vi "Create or Close PDFReader.vi"(2 "Action":T1, 5 "PdfReader IN":refnum<k24>, 7 "PDF File and position":T2={"Path"=path "", "Pages"="all", "Source"=enum."File to add", "Start at page old"=0, "Start at page new"=1, "Owner password"=""}, 11 "error in (no error)":errorcluster) -> (4 "PDFReaderIsOpen?":bool, 6 "PdfReader OUT":refnum<k24>, 8 "NumberOfPages":i32, 10 "Page [ ]":i32[](array[numeric]), 15 "error out":errorcluster)   [LabVIEW 2019, in "Exaprom PDF.lvlib"]
doc: "Version 1.1\nDeveloped by Jean-Marc Simard\nCopyright © 2012, Exaprom Inc.\nAll rights reserved.\nLicense: BSD\n\nWith iTextSharp 4.1.6 (http://itextsharp.sourceforge.net)\nunder Mozilla Public License Version 1.1\n(http://www.mozilla.org/MPL/MPL-1.1.html)"
uses:
  Controls/Concatenate Controls/PDF File and position.ctl
  Controls/Concatenate Controls/PDF file source.ctl
  C:/work/niobrara_lv/labview pdf writer fixing/DLL/itextsharp.dll
  DLL/itextsharp.dll
  Controls/General Controls/Create or close.ctl
  Exaprom PDF.lvlib
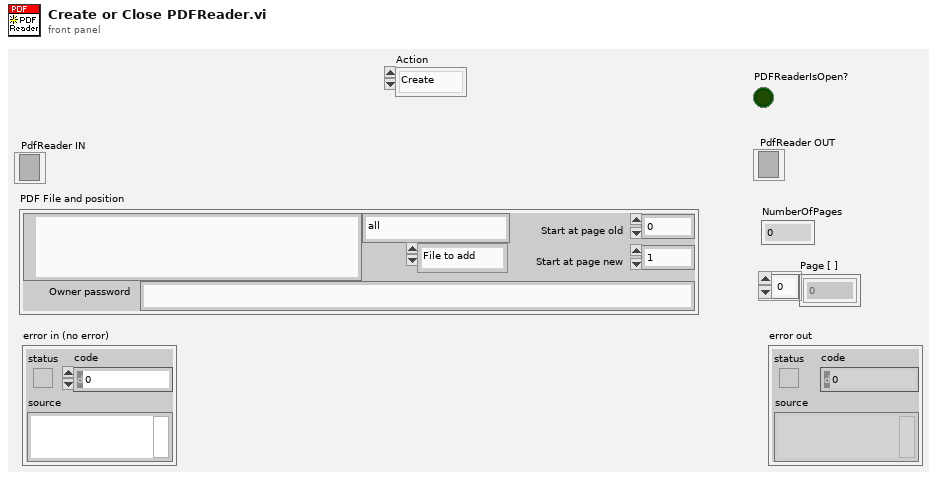
[diagram p1: front panel]
types:
  T1 = typedef "Exaprom PDF.lvlib/Create or close.ctl" = enum16{"Create", "Close"}
  T2 = typedef "Exaprom PDF.lvlib/PDF File and position.ctl" = cluster{"Path":path, "Pages":string, "Source":T3, "Start at page old":i32, "Start at page new":i32, "Owner password":string}
  T3 = typedef "Exaprom PDF.lvlib/PDF file source.ctl" = enum16{"PDF Report", "File to add"}
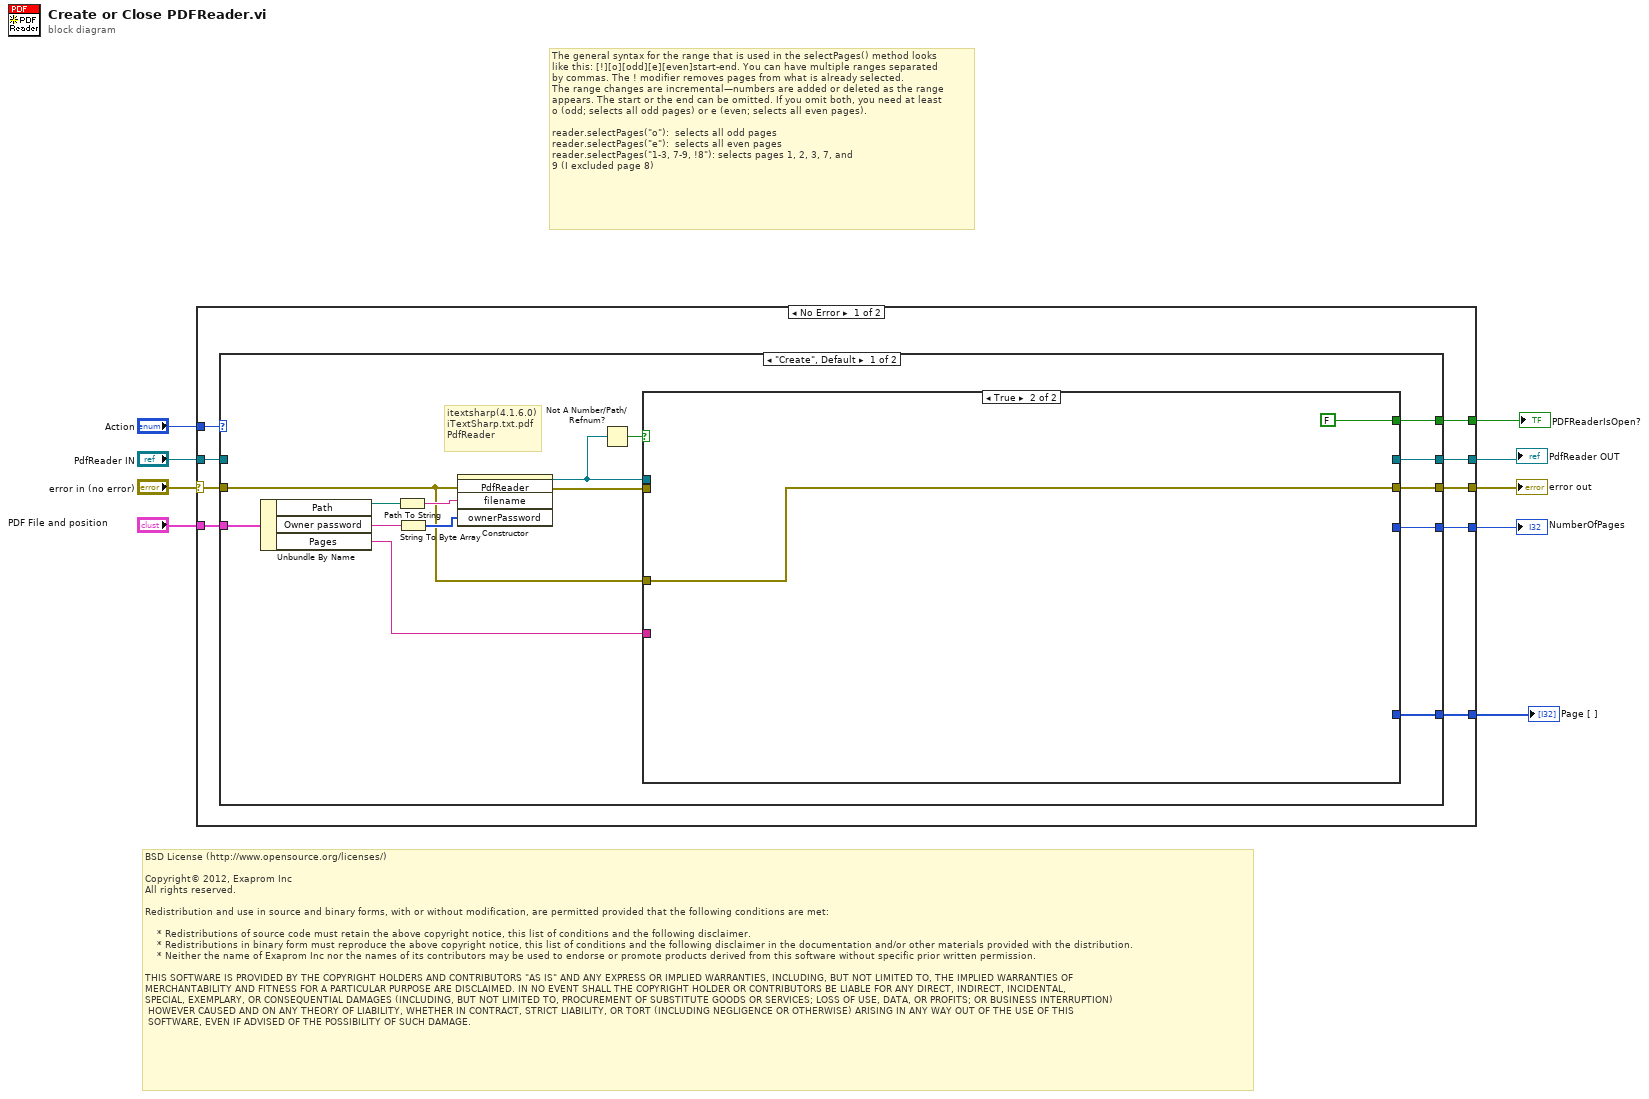
[diagram p0: block diagram]
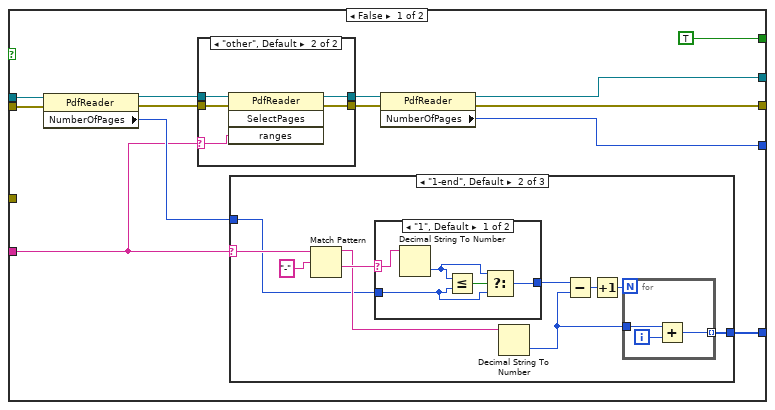
[diagram p2: hidden frame]
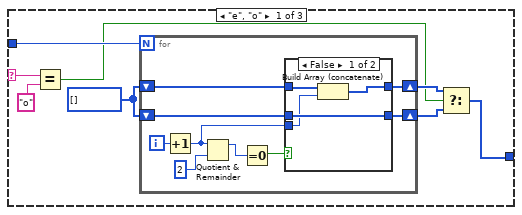
[diagram p3: hidden frame]
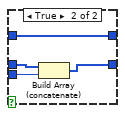
[diagram p4: hidden frame]
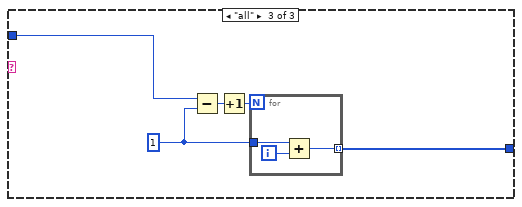
[diagram p6: hidden frame]
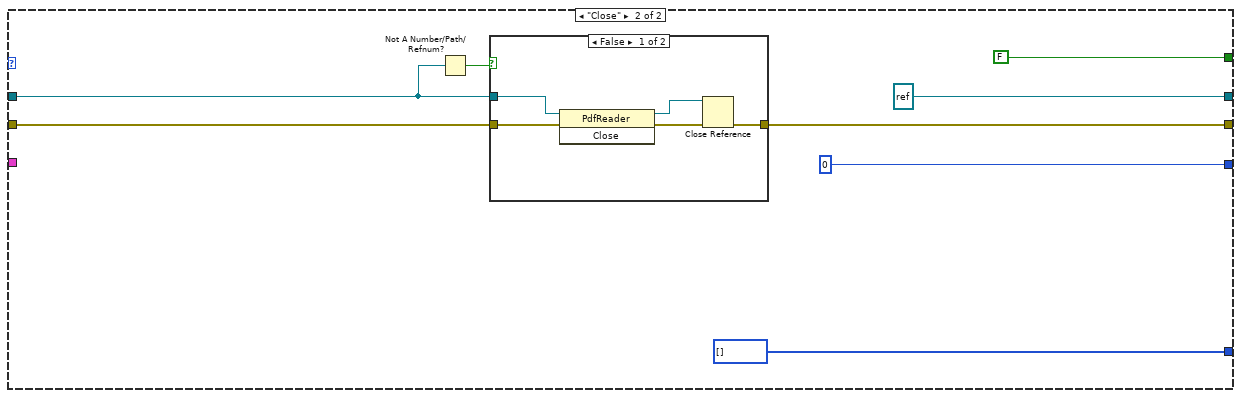
[diagram p8: hidden frame]
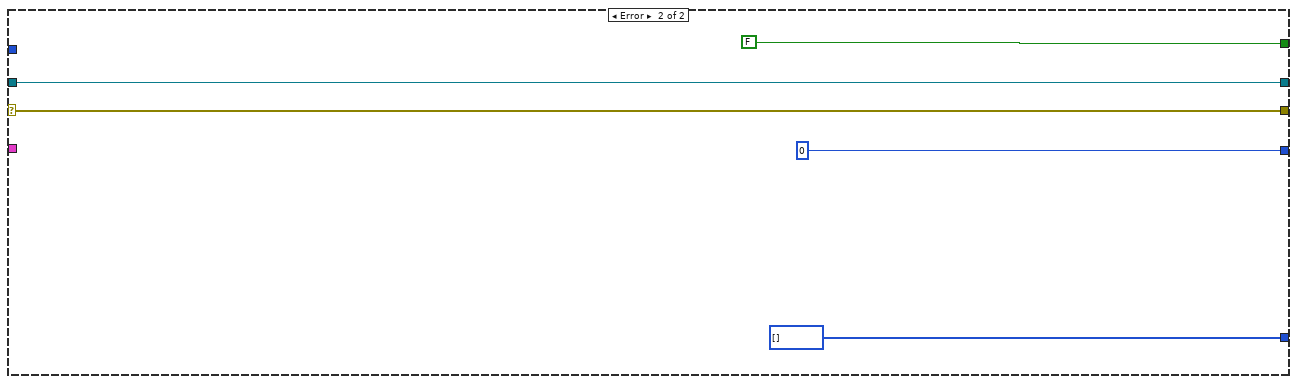
[diagram p10: hidden frame]
diagram:
  # "The general syntax for the range that is used in the selectPages() method looks\nlike this: [!][o][odd][e][even]start-end. You can have multiple ranges separated\nby commas. The ! modifier removes pages from what is already selected.\nThe range changes are incremental—numbers are added or deleted as the range\nappears. The start or the end can be omitted. If you omit both, you need at least\no (odd; selects all odd pages) or e (even; selects all even pages).\n\nreader.selectPages(\"o\"):  selects all odd pages\nreader.selectPages(\"e\"):  selects all even pages\nreader.selectPages(\"1-3, 7-9, !8\"): selects pages 1, 2, 3, 7, and\n9 (I excluded page 8)"
  # "BSD License (http://www.opensource.org/licenses/)\n\nCopyright© 2012, Exaprom Inc\nAll rights reserved.\n\nRedistribution and use in source and binary forms, with or without modification, are permitted provided that the following conditions are met:\n\n    * Redistributions of source code must retain the above copyright notice, this list of conditions and the following disclaimer.\n    * Redistributions in binary form must reproduce the above copyright notice, this list of conditions and the following disclaimer in the documentation and/or other materials provided with the distribution.\n    * Neither the name of Exaprom Inc nor the names of its contributors may be used to endorse or promote products derived from this software without specific prior written permission.\n\nTHIS SOFTWARE IS PROVIDED BY THE COPYRIGHT HOLDERS AND CONTRIBUTORS \"AS IS\" AND ANY EXPRESS OR IMPLIED WARRANTIES, INCLUDING, BUT NOT LIMITED TO, THE IMPLIED WARRANTIES OF \nMERCHANTABILITY AND FITNESS FOR A PARTICULAR PURPOSE ARE DISCLAIMED. IN NO EVENT SHALL THE COPYRIGHT HOLDER OR CONTRIBUTORS BE LIABLE FOR ANY DIRECT, INDIRECT, INCIDENTAL,\nSPECIAL, EXEMPLARY, OR CONSEQUENTIAL DAMAGES (INCLUDING, BUT NOT LIMITED TO, PROCUREMENT OF SUBSTITUTE GOODS OR SERVICES; LOSS OF USE, DATA, OR PROFITS; OR BUSINESS INTERRUPTION)\n HOWEVER CAUSED AND ON ANY THEORY OF LIABILITY, WHETHER IN CONTRACT, STRICT LIABILITY, OR TORT (INCLUDING NEGLIGENCE OR OTHERWISE) ARISING IN ANY WAY OUT OF THE USE OF THIS\n SOFTWARE, EVEN IF ADVISED OF THE POSSIBILITY OF SUCH DAMAGE."
  n1 = case shown="No Error" "error in (no error)" {
    selector: "error in (no error)" -> [w17 w126]
    tunnel: [w16 w126] -> w9
    tunnel: "PDF File and position" -> [w18 _]
    tunnel: [w15 w125] -> w5
    tunnel: [w14 0 ("NumberOfPages")] -> w6
    tunnel: "Action" -> [w13 _]
    tunnel: "PdfReader IN" -> [w12 w125]
    tunnel: [w11 i32[] []] -> w2
    tunnel: [w10 FALSE] -> w1
    frame No Error {
      n2 = case shown="\"Create\", Default" w13 {
        tunnel: w18 -> [w27 _]
        tunnel: w17 -> [w19 w115]
        tunnel: [w32 w113] -> w16
        tunnel: [w31 refnum<k24> refnum ("new reference")] -> w15
        tunnel: [w30 0 ("NumberOfPages")] -> w14
        tunnel: w12 -> [_ w108]
        tunnel: [w28 i32[] []] -> w11
        tunnel: [w20 FALSE] -> w10
        frame "Create", Default {
          # "itextsharp(4.1.6.0)\niTextSharp.txt.pdf\nPdfReader"
          n3 = Unbundle By Name(w27) -> ("Path"=w26:path, "Owner password"=w25:string, "Pages"=w24:string)
          n4 = Path To String(path=w26) -> (string=w33:string)
          n5 = String To Byte Array(string=w25) -> (unsigned byte array=w23:u8[])
          n6 = constructor class="PdfReader"(error in=w19, "filename"=w33, "ownerPassword"=w23) -> (reference out=w21:refnum<k24>, error out=w29:errorcluster)  [unwired: 2 in, 3 out]
          n7 = Not A Number/Path/Refnum?(number/path/refnum=w21) -> (NaN/Path/Refnum?=w22:bool)
          n8 = case shown="True" w22 {
            tunnel: [w44 w106] -> w32
            tunnel: [w43 _] -> w31
            tunnel: [w42 _] -> w30
            tunnel: w29 -> [w39 _]
            tunnel: [w37 _] -> w28
            tunnel: w21 -> [w36 _]
            tunnel: w24 -> [w35 _]
            tunnel: [TRUE FALSE] -> w20
            tunnel: w19 -> [_ w106]
            frame False {
              n9 = property class="PdfReader"(reference=w36, error in=w39) -> (reference out=w41:refnum<k24>, error out=w40:errorcluster, "NumberOfPages"=w38:i32)
              n10 = case shown="\"other\", Default" w35 {
                selector: w35 -> [_ w101]
                tunnel: w41 -> [w100 w105]
                tunnel: w40 -> [w99 w104]
                tunnel: [w99 w103] -> w46
                tunnel: [w100 w102] -> w45
                frame "all" {
                }
                frame "other", Default {
                  n11 = invoke class="PdfReader" method="SelectPages"(reference=w105, error in=w104, "ranges"=w101) -> (reference out=w102:refnum<k24>, error out=w103:errorcluster)  [unwired: 1 in, 2 out]
                }
              }
              n12 = case shown="\"1-end\", Default" w35 {
                selector: w35 -> [w49 w74 _]
                tunnel: w38 -> [w53 w73 w92]
                tunnel: [w50 w72 w93] -> w37
                frame "e", "o" {
                  w54 = i32[] []
                  n13 = Equal?(x=w49, y="o") -> (x = y?=w47:bool)
                  n14 = for {
                    N: w53 -> [_]
                    shift-right: [w60] -> w52
                    shift-left: w54 -> [w59]
                    shift-right: [w57] -> w51
                    shift-left: w54 -> [w58]
                    i -> [w63]
                    n15 = Increment(x=w63) -> (x+1=w56:i32)
                    n16 = Quotient & Remainder(x=w56, y=2) -> (x-y*floor(x/y)=w55:i32)  [unwired: 1 out]
                    n17 = Equal To 0?(x=w55) -> (x = 0?=w61:bool)
                    n18 = case shown="False" w61 {
                      tunnel: [w65 w71] -> w60
                      tunnel: w59 -> [w66 w71]
                      tunnel: w58 -> [w67 w70]
                      tunnel: [w67 w69] -> w57
                      tunnel: w56 -> [w64 w68]
                      frame False {
                        n19 = Build Array (concatenate)(w66, w64) -> (w65:i32[])
                      }
                      frame True {
                        n20 = Build Array (concatenate)(w70, w68) -> (w69:i32[])
                      }
                    }
                  }
                  n21 = Select(t=w52, s=w47, f=w51) -> (s? t:f=w50:i32[])
                }
                frame "1-end", Default {
                  n22 = Match Pattern(string=w74, regular expression="-") -> (before substring=w79:string, after substring=w80:string)  [unwired: 1 in, 2 out]
                  n23 = case shown="\"1\", Default" w80 {
                    selector: w80 -> [w89 _]
                    tunnel: w73 -> [w86 w90]
                    tunnel: [w85 w90] -> w78
                    frame "1", Default {
                      n24 = Decimal String To Number(string=w89) -> (number=w87:i32)  [unwired: 2 in, 1 out]
                      n25 = Less Or Equal?(x=w87, y=w86) -> (x <= y?=w88:bool)
                      n26 = Select(t=w87, s=w88, f=w86) -> (s? t:f=w85:i32)
                    }
                    frame "end" {
                    }
                  }
                  n27 = Decimal String To Number(string=w79) -> (number=w76:i32)  [unwired: 2 in, 1 out]
                  n28 = Subtract(x=w78, y=w76) -> (x-y=w77:i32)
                  n29 = Increment(x=w77) -> (x+1=w75:i32)
                  n30 = for {
                    N: w75 -> [_]
                    tunnel: w76 -> [w84]
                    tunnel: [w82] -> w72 mode=indexing
                    i -> [w83]
                    n31 = Add(x=w84, y=w83) -> (x+y=w82:i32)
                  }
                }
                frame "all" {
                  w91 = 1 ("y")
                  n32 = Subtract(x=w92, y=w91) -> (x-y=w95:i32)
                  n33 = Increment(x=w95) -> (x+1=w94:i32)
                  n34 = for {
                    N: w94 -> [_]
                    tunnel: w91 -> [w98]
                    tunnel: [w96] -> w93 mode=indexing
                    i -> [w97]
                    n35 = Add(x=w98, y=w97) -> (x+y=w96:i32)
                  }
                }
              }
              n36 = property class="PdfReader"(reference=w45, error in=w46) -> (reference out=w43:refnum<k24>, error out=w44:errorcluster, "NumberOfPages"=w42:i32)
            }
            frame True {
            }
          }
        }
        frame "Close" {
          n37 = Not A Number/Path/Refnum?(number/path/refnum=w108) -> (NaN/Path/Refnum?=w109:bool)
          n38 = case shown="False" w109 {
            tunnel: w115 -> [w120 w121]
            tunnel: w108 -> [w118 _]
            tunnel: [w117 w121] -> w113
            frame False {
              n39 = invoke class="PdfReader" method="Close"(reference=w118, error in=w120) -> (reference out=w116:refnum<k24>, error out=w119:errorcluster)  [unwired: 1 in, 1 out]
              n40 = Close Reference(reference=w116, error in (no error)=w119) -> (error out=w117:errorcluster)
            }
            frame True {
            }
          }
        }
      }
    }
    frame Error {
    }
  }
  "error out" <- w9
  "NumberOfPages" <- w6
  "PdfReader OUT" <- w5
  "Page [ ]" <- w2
  "PDFReaderIsOpen?" <- w1
